vi "DrawJoystick.vi"(11 "Joystick":T2) -> (3 "DrawJoy":T1 {"Slide" scale=-1.0..1.0; "Trigger" scale=-1.0..1.0})   [LabVIEW 2012]
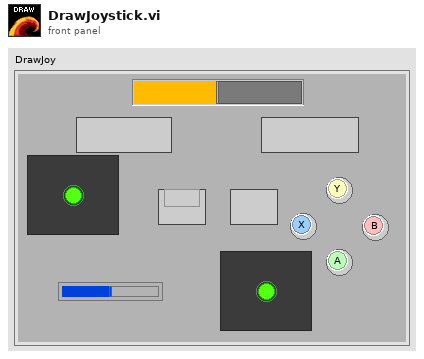
[diagram p1: front panel]
types:
  T1 = cluster{"Y":bool, "B":bool, "X":bool, "A":bool, "Left Bumper":bool, "Right Bumper":bool, "Joystick 2":cluster{"X":dbl, "Y":dbl}[], "Joystick 3":cluster{"X":dbl, "Y":dbl}[], "Back":bool, "Start":bool, "Trigger":dbl, "Slide":dbl, "Left Thumbstick":bool, "Right Thumbstick":bool}
  T2 = cluster{"Buttons":cluster{"A":bool, "B":bool, "X":bool, "Y":bool, "Left Bumper":bool, "Right Bumper":bool, "Back":bool, "Start":bool, "Left Thumbstick":bool, "Right Thumbstick":bool}, "Axes":cluster{"Left Stick X ":dbl, "Left Stick Y":dbl, "Triggers":dbl, "Right Stick X":dbl, "Right Stick Y":dbl, "D-Pad X":dbl}}
  T3 = cluster{"Right Stick X":dbl, "Right Stick Y":dbl}
  T4 = cluster{"Left Stick X ":dbl, "Left Stick Y":dbl}[]
  T5 = cluster{"Right Stick X":dbl, "Right Stick Y":dbl}[]
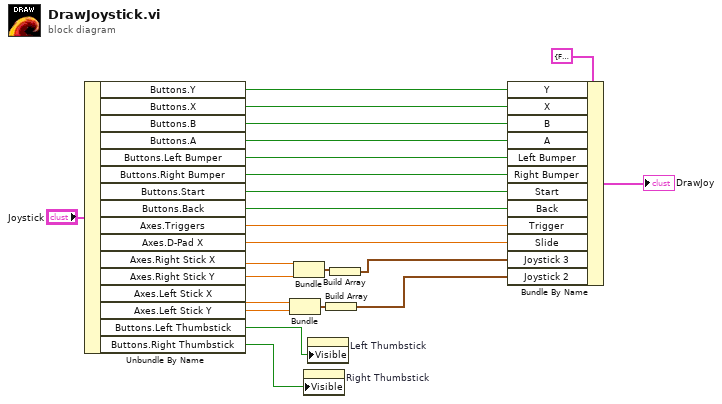
[diagram p0: block diagram]
diagram:
  n1 = Unbundle By Name("Joystick") -> ("Buttons.Y"=w16:bool, "Buttons.X"=w15:bool, "Buttons.B"=w14:bool, "Buttons.A"=w13:bool, "Buttons.Left Bumper"=w12:bool, "Buttons.Right Bumper"=w11:bool, "Buttons.Start"=w10:bool, "Buttons.Back"=w9:bool, "Axes.Triggers"=w8:dbl, "Axes.D-Pad X"=w7:dbl, "Axes.Right Stick X"=w6:dbl, "Axes.Right Stick Y"=w5:dbl, "Axes.Left Stick X"=w21:dbl, "Axes.Left Stick Y"=w20:dbl, "Buttons.Left Thumbstick"=w2:bool, "Buttons.Right Thumbstick"=w1:bool)
  n2 = Bundle("Left Stick X"=w21, "Left Stick Y"=w20) -> (w23:cluster{"Left Stick X ":dbl, "Left Stick Y":dbl})  [unwired: 1 in]
  n3 = Bundle("Right Stick X"=w6, "Right Stick Y"=w5) -> (w22:T3)  [unwired: 1 in]
  n4 = property on="Right Thumbstick" class="Bool (strict)"("Visible"=w1) -> ()  [unwired: 2 in, 2 out]
  n5 = property on="Left Thumbstick" class="Bool (strict)"("Visible"=w2) -> ()  [unwired: 2 in, 2 out]
  n6 = Build Array(w23) -> (w3:T4)
  n7 = Build Array(w22) -> (w4:T5)
  n8 = Bundle By Name(cluster=T1 {"Y"=FALSE, "B"=FALSE, "X"=FALSE, "A"=FALSE, "Left Bumper"=FALSE, "Right Bumper"=FALSE, "Joystick 2"=[], "Joystick 3"=[], "Back"=FALSE, "Start"=FALSE, "Trigger"=0.0, "Slide"=0.0, "Left Thumbstick"=FALSE, "Right Thumbstick"=TRUE} ("DrawJoy"), "Y"=w16, "X"=w15, "B"=w14, "A"=w13, "Left Bumper"=w12, "Right Bumper"=w11, "Start"=w10, "Back"=w9, "Trigger"=w8, "Slide"=w7, "Joystick 3"=w4, "Joystick 2"=w3) -> (→"DrawJoy":T1)
